vi "Read Position.vi"(8 "error in (no error)":errorcluster, 11 "window in":refnum<class "window.lvclass">) -> (0 "error out":errorcluster, 2 "Position":T1, 3 "window out":refnum<class "window.lvclass">)   [LabVIEW 2013, in "frontPanelObjects.lvlib" / "window.lvclass"]
uses:
  window.lvclass
  <vilib>/Utility/miscctls.llb/LVPositionTypeDef.ctl
  window.lvclass/window.ctl
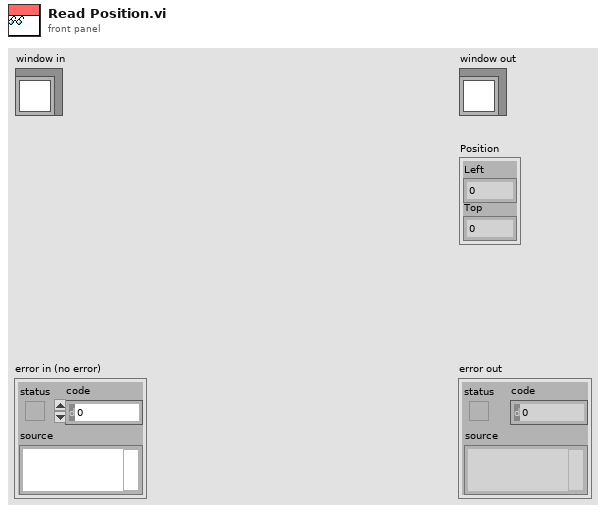
[diagram p1: front panel]
types:
  T1 = typedef "LVPositionTypeDef.ctl" = cluster{"Left":i32, "Top":i32}
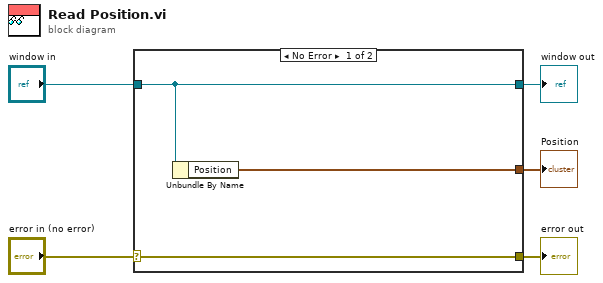
[diagram p0: block diagram]
diagram:
  n1 = case shown="No Error" "error in (no error)" {
    selector: "error in (no error)" -> [w8 w9]
    tunnel: [w8 w9] -> w4
    tunnel: [w7 w10] -> w2
    tunnel: "window in" -> [w7 w10]
    tunnel: [w6 _] -> w1
    frame No Error {
      n2 = Unbundle By Name(w7) -> ("Position"=w6:T1)
    }
    frame Error {
    }
  }
  "error out" <- w4
  "window out" <- w2
  "Position" <- w1
